vi "Tx Disable channel logic 4ch 4SPC.vi"(5 "num channels":u32, 6 "ready for output":bool, 9 "input valid":bool, 10 "data in":u32[](array[numeric])=[0, 0, 0, 0, 0, 0, 0, 0, 0, 0, 0, 0, 0, 0, 0, 0], 11 "enabled channels":u32) -> (0 "enable new data":bool, 1 "output valid":bool, 2 "data out":u32[](array[numeric]))   [LabVIEW 2025, in "niUSRP Stream Control (DMA) v1 FPGA.lvclass"]
uses:
  niUSRP Stream Control (DMA) v1 FPGA.lvclass
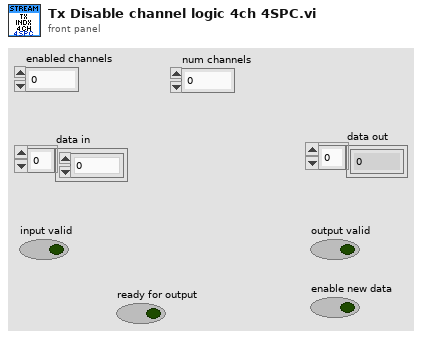
[diagram p1: front panel]
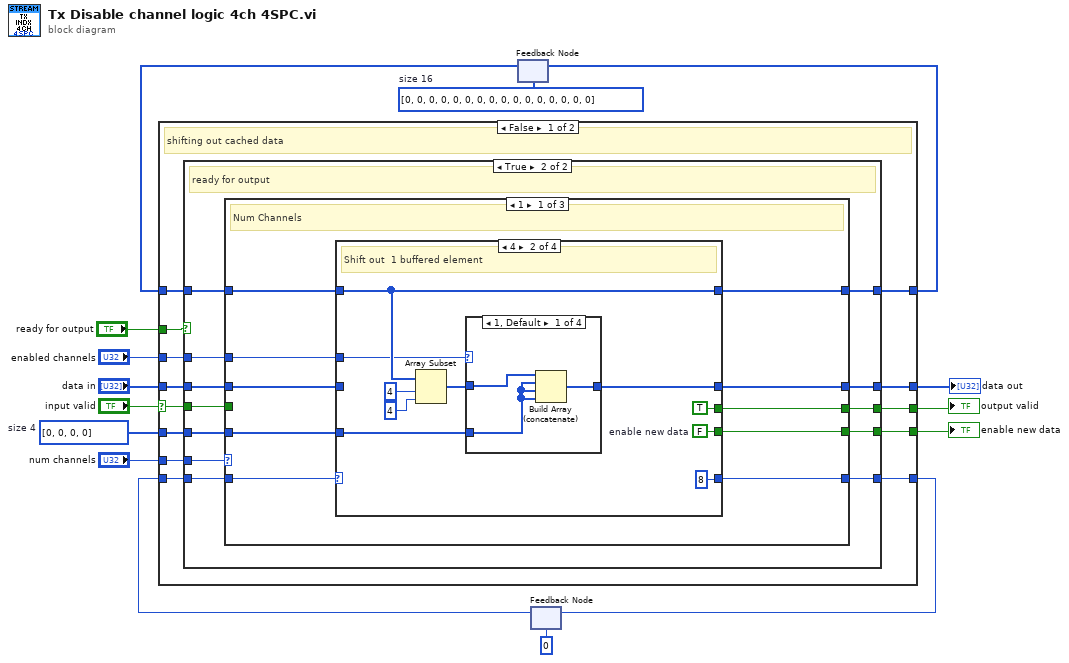
[diagram p0: block diagram]
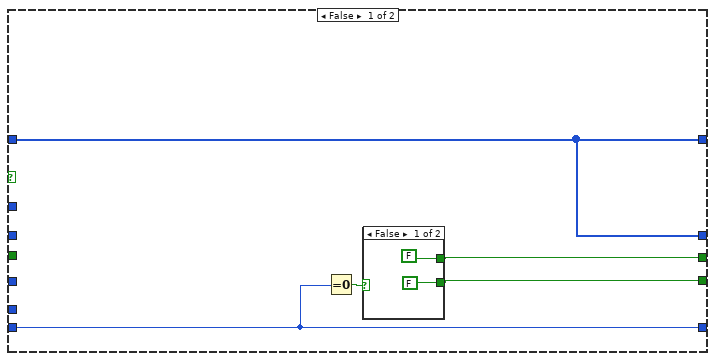
[diagram p2: hidden frame]
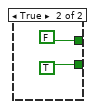
[diagram p3: hidden frame]
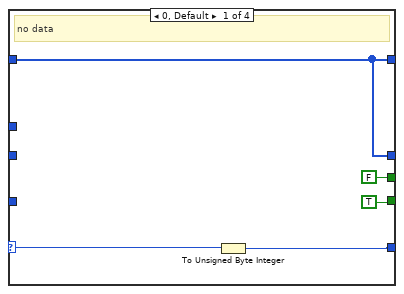
[diagram p4: hidden frame]
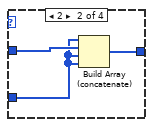
[diagram p5: hidden frame]
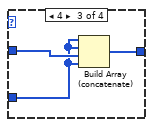
[diagram p6: hidden frame]
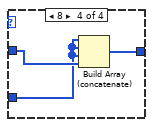
[diagram p7: hidden frame]
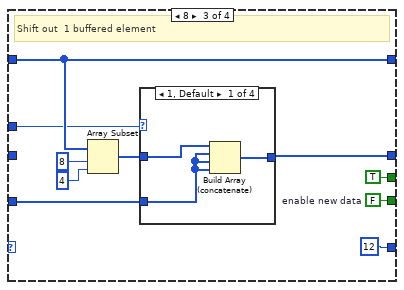
[diagram p8: hidden frame]
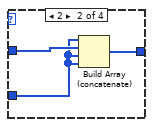
[diagram p9: hidden frame]
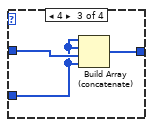
[diagram p10: hidden frame]
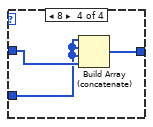
[diagram p11: hidden frame]
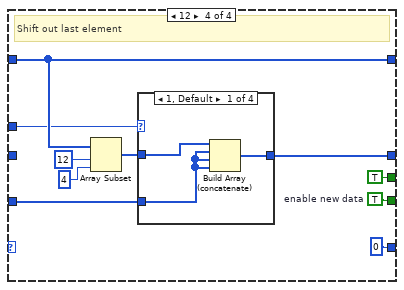
[diagram p12: hidden frame]
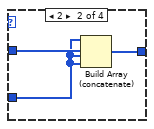
[diagram p13: hidden frame]
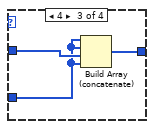
[diagram p14: hidden frame]
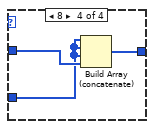
[diagram p15: hidden frame]
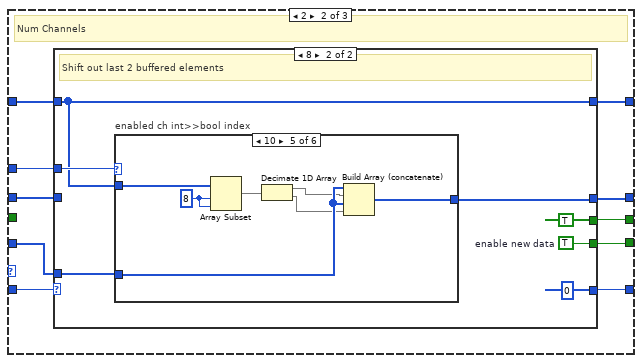
[diagram p16: hidden frame]
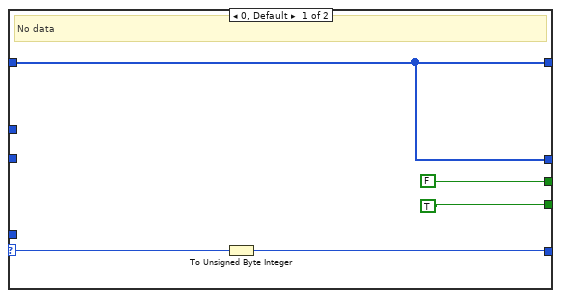
[diagram p17: hidden frame]
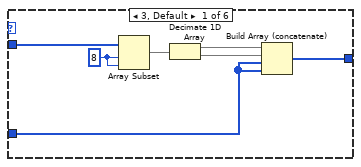
[diagram p18: hidden frame]
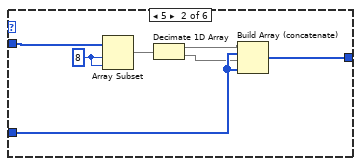
[diagram p19: hidden frame]
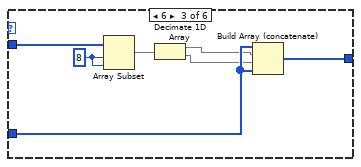
[diagram p20: hidden frame]
diagram:
  w2 = u32[] [0, 0, 0, 0]  # size 4
  w7 = u32[] [0, 0, 0, 0, 0, 0, 0, 0, 0, 0, 0, 0, 0, 0, 0, 0]  # size 16
  n1 = feedback #1(w7) -> (w6:u32[])
  n2 = feedback #2(u8 0) -> (w3:u8)
  n3 = case shown="False" "input valid" {
    selector: "input valid" -> [w19 _]
    tunnel: "num channels" -> [w28 w211]
    tunnel: [w27 w207] -> w14
    tunnel: [w26 w206] -> w13
    tunnel: "data in" -> [w25 w208]
    tunnel: "enabled channels" -> [w24 w203]
    tunnel: [w23 w205] -> w10
    tunnel: w6 -> [w22 w202]
    tunnel: [w21 w204] -> w5
    tunnel: [w16 w210] -> w4
    tunnel: w3 -> [w20 w209]
    tunnel: w2 -> [w18 w201]
    tunnel: "ready for output" -> [w17 _]
    frame False {
      # "shifting out cached data"
      n4 = case shown="True" w17 {
        tunnel: w28 -> [_ w49]
        tunnel: [w31 w48] -> w27
        tunnel: [w30 w47] -> w26
        tunnel: w25 -> [_ w46]
        tunnel: w24 -> [_ w45]
        tunnel: [w29 w44] -> w23
        tunnel: w22 -> [w29 w43]
        tunnel: [w29 w42] -> w21
        tunnel: w20 -> [w32 w41]
        tunnel: w19 -> [_ w39]
        tunnel: w18 -> [_ w38]
        tunnel: [w32 w40] -> w16
        frame False {
          n5 = Equal To 0?(x=w32) -> (x = 0?=w33:bool)
          n6 = case shown="False" w33 {
            tunnel: [FALSE TRUE] -> w30
            tunnel: [FALSE FALSE] -> w31
            frame False {
            }
            frame True {
            }
          }
        }
        frame True {
          # "ready for output"
          n7 = case shown="1" w49 {
            tunnel: w45 -> [w59 w139 _]
            tunnel: w46 -> [w58 w140 w200]
            tunnel: [w57 w136 w199] -> w47
            tunnel: [w56 w137 w196] -> w48
            tunnel: [w55 w138 w200] -> w44
            tunnel: w43 -> [w51 w132 w197]
            tunnel: [w54 w133 w197] -> w42
            tunnel: w41 -> [w53 w134 w198]
            tunnel: [w52 w135 w195] -> w40
            tunnel: w39 -> [_ _ w196]
            tunnel: w38 -> [w50 w131 _]
            frame 1 {
              # "Num Channels"
              n8 = case shown="4" w53 {
                selector: w53 -> [w61 _ _ _]
                tunnel: w58 -> [_ _ _ _]
                tunnel: [w60 u8 8 ("length") u8 12 ("length") u8 0] -> w52
                tunnel: [w62 w65 w96 w113] -> w55
                tunnel: [FALSE TRUE TRUE TRUE] -> w56
                tunnel: w51 -> [w62 w73 w94 w115]
                tunnel: [w62 w73 w94 w115] -> w54
                tunnel: [TRUE w72 w93 w116] -> w57
                tunnel: w59 -> [_ w67 w92 w112]
                tunnel: w50 -> [_ w68 w90 w111]
                frame 0, Default {
                  # "no data"
                  n9 = To Unsigned Byte Integer(number=w61) -> (unsigned 8bit integer=w60:u8)
                }
                frame 4 {
                  w72 = FALSE  # enable new data
                  # "Shift out  1 buffered element"
                  n10 = Array Subset(array=w73, index=i16 4 ("length"), length=i16 4) -> (w66:u32[])
                  n11 = case shown="1, Default" w67 {
                    tunnel: [w77 w80 w83 w86] -> w65
                    tunnel: w66 -> [w76 w79 w82 w85]
                    tunnel: w68 -> [w75 w78 w81 w84]
                    frame 1, Default {
                      n12 = Build Array (concatenate)(w76, w75, w75, w75) -> (w77:u32[])
                    }
                    frame 2 {
                      n13 = Build Array (concatenate)(w78, w79, w78, w78) -> (w80:u32[])
                    }
                    frame 4 {
                      n14 = Build Array (concatenate)(w81, w81, w82, w81) -> (w83:u32[])
                    }
                    frame 8 {
                      n15 = Build Array (concatenate)(w84, w84, w84, w85) -> (w86:u32[])
                    }
                  }
                }
                frame 8 {
                  w93 = FALSE  # enable new data
                  # "Shift out  1 buffered element"
                  n16 = Array Subset(array=w94, index=i16 8 ("length"), length=i16 4) -> (w91:u32[])
                  n17 = case shown="1, Default" w92 {
                    tunnel: [w99 w102 w105 w108] -> w96
                    tunnel: w91 -> [w98 w101 w104 w107]
                    tunnel: w90 -> [w97 w100 w103 w106]
                    frame 1, Default {
                      n18 = Build Array (concatenate)(w98, w97, w97, w97) -> (w99:u32[])
                    }
                    frame 2 {
                      n19 = Build Array (concatenate)(w100, w101, w100, w100) -> (w102:u32[])
                    }
                    frame 4 {
                      n20 = Build Array (concatenate)(w103, w103, w104, w103) -> (w105:u32[])
                    }
                    frame 8 {
                      n21 = Build Array (concatenate)(w106, w106, w106, w107) -> (w108:u32[])
                    }
                  }
                }
                frame 12 {
                  w116 = TRUE  # enable new data
                  # "Shift out last element"
                  n22 = Array Subset(array=w115, index=12, length=4) -> (w109:u32[])
                  n23 = case shown="1, Default" w112 {
                    tunnel: [w121 w124 w127 w130] -> w113
                    tunnel: w109 -> [w120 w123 w126 w129]
                    tunnel: w111 -> [w119 w122 w125 w128]
                    frame 1, Default {
                      n24 = Build Array (concatenate)(w120, w119, w119, w119) -> (w121:u32[])
                    }
                    frame 2 {
                      n25 = Build Array (concatenate)(w122, w123, w122, w122) -> (w124:u32[])
                    }
                    frame 4 {
                      n26 = Build Array (concatenate)(w125, w125, w126, w125) -> (w127:u32[])
                    }
                    frame 8 {
                      n27 = Build Array (concatenate)(w128, w128, w128, w129) -> (w130:u32[])
                    }
                  }
                }
              }
            }
            frame 2 {
              # "Num Channels"
              n28 = case shown="8" w134 {
                selector: w134 -> [w142 _]
                tunnel: w140 -> [_ _]
                tunnel: [w141 u8 0] -> w135
                tunnel: [w143 w148] -> w138
                tunnel: [FALSE TRUE] -> w137
                tunnel: w132 -> [w143 w146]
                tunnel: [w143 w146] -> w133
                tunnel: [TRUE w150] -> w136
                tunnel: w139 -> [_ w149]
                tunnel: w131 -> [_ w147]
                frame 0, Default {
                  # "No data"
                  n29 = To Unsigned Byte Integer(number=w142) -> (unsigned 8bit integer=w141:u8)
                }
                frame 8 {
                  w150 = TRUE  # enable new data
                  # "Shift out last 2 buffered elements"
                  n30 = case "enabled ch int>>bool index" shown="10" w149 {
                    tunnel: [w159 w166 w173 w180 w187 w194] -> w148
                    tunnel: w147 -> [w158 w165 w172 w179 w186 w193]
                    tunnel: w146 -> [w156 w162 w169 w176 w183 w190]
                    frame 3, Default {
                      w155 = 8 ("index")
                      n31 = Array Subset(array=w156, index=w155, length=w155) -> (w157:u32[])
                      n32 = Decimate 1D Array(w157) -> (w154:u32[], w153:u32[])
                      n33 = Build Array (concatenate)(w154, w153, w158, w158) -> (w159:u32[])
                    }
                    frame 5 {
                      w163 = 8 ("index")
                      n34 = Array Subset(array=w162, index=w163, length=w163) -> (w164:u32[])
                      n35 = Decimate 1D Array(w164) -> (w161:u32[], w160:u32[])
                      n36 = Build Array (concatenate)(w161, w165, w160, w165) -> (w166:u32[])
                    }
                    frame 6 {
                      w170 = 8 ("index")
                      n37 = Array Subset(array=w169, index=w170, length=w170) -> (w171:u32[])
                      n38 = Decimate 1D Array(w171) -> (w168:u32[], w167:u32[])
                      n39 = Build Array (concatenate)(w172, w168, w167, w172) -> (w173:u32[])
                    }
                    frame 9 {
                      w177 = 8 ("index")
                      n40 = Array Subset(array=w176, index=w177, length=w177) -> (w178:u32[])
                      n41 = Decimate 1D Array(w178) -> (w175:u32[], w174:u32[])
                      n42 = Build Array (concatenate)(w175, w179, w179, w174) -> (w180:u32[])
                    }
                    frame 10 {
                      w184 = 8 ("index")
                      n43 = Array Subset(array=w183, index=w184, length=w184) -> (w185:u32[])
                      n44 = Decimate 1D Array(w185) -> (w182:u32[], w181:u32[])
                      n45 = Build Array (concatenate)(w186, w182, w186, w181) -> (w187:u32[])
                    }
                    frame 12 {
                      w191 = 8 ("index")
                      n46 = Array Subset(array=w190, index=w191, length=w191) -> (w192:u32[])
                      n47 = Decimate 1D Array(w192) -> (w189:u32[], w188:u32[])
                      n48 = Build Array (concatenate)(w193, w193, w189, w188) -> (w194:u32[])
                    }
                  }
                }
              }
            }
            frame 4, Default {
              w199 = TRUE  # enable new data
              # "Num Channels"
              n49 = To Unsigned Byte Integer(number=w198) -> (unsigned 8bit integer=w195:u8)
            }
          }
        }
      }
    }
    frame True {
      # "input valid >>cache data"
      n50 = case shown="1, Default" w211 {
        tunnel: [u8 4 ("x") u8 8 ("length") u8 0 ("length")] -> w210
        tunnel: w209 -> [_ _ _]
        tunnel: w208 -> [w217 w234 w290]
        tunnel: [TRUE TRUE TRUE] -> w207
        tunnel: [w220 FALSE ("enable new data") w297] -> w206
        tunnel: [w212 w235 w289] -> w205
        tunnel: [w217 w234 w295] -> w204
        tunnel: w203 -> [w215 w237 _]
        tunnel: w202 -> [_ _ w295]
        tunnel: w201 -> [w213 w236 _]
        frame 1, Default {
          w220 = FALSE  # enable new data
          # "Send data to enabled channel\nRemaining 3 channels set to default \"0\""
          # "Grab data for \n1ch - 4SPC"
          # "Num Enabled Channels"
          n51 = Array Subset(array=w217, index=0, length=4) -> (w214:u32[])
          n52 = case shown="1, Default" w215 {
            tunnel: [w224 w227 w230 w233] -> w212
            tunnel: w213 -> [w223 w226 w229 w232]
            tunnel: w214 -> [w222 w225 w228 w231]
            frame 1, Default {
              # "enabled ch int>>bool index"
              n53 = Build Array (concatenate)(w222, w223, w223, w223) -> (w224:u32[])
            }
            frame 2 {
              # "enabled ch int>>bool index"
              n54 = Build Array (concatenate)(w226, w225, w226, w226) -> (w227:u32[])
            }
            frame 4 {
              # "enabled ch int>>bool index"
              n55 = Build Array (concatenate)(w229, w229, w228, w229) -> (w230:u32[])
            }
            frame 8 {
              # "enabled ch int>>bool index"
              n56 = Build Array (concatenate)(w232, w232, w232, w231) -> (w233:u32[])
            }
          }
        }
        frame 2 {
          # "Grab 2 channels\ninterleaved data\n(0,1,0,1,0,1,0,1..)"
          # "Num Enabled Channels"
          n57 = case "enabled ch int>>bool index" shown="3, Default" w237 {
            tunnel: [w248 w256 w264 w272 w280 w288] -> w235
            tunnel: w236 -> [w247 w255 w263 w271 w279 w287]
            tunnel: w234 -> [w245 w251 w259 w267 w275 w283]
            frame 3, Default {
              n58 = Array Subset(array=w245, index=0 ("y"), length=8 ("y")) -> (w246:u32[])
              n59 = Decimate 1D Array(w246) -> (w242:u32[], w241:u32[])
              n60 = Build Array (concatenate)(w242, w241, w247, w247) -> (w248:u32[])
            }
            frame 5 {
              n61 = Array Subset(array=w251, index=0 ("y"), length=8 ("y")) -> (w254:u32[])
              n62 = Decimate 1D Array(w254) -> (w250:u32[], w249:u32[])
              n63 = Build Array (concatenate)(w250, w255, w249, w255) -> (w256:u32[])
            }
            frame 6 {
              n64 = Array Subset(array=w259, index=0 ("y"), length=8 ("y")) -> (w262:u32[])
              n65 = Decimate 1D Array(w262) -> (w258:u32[], w257:u32[])
              n66 = Build Array (concatenate)(w263, w258, w257, w263) -> (w264:u32[])
            }
            frame 9 {
              n67 = Array Subset(array=w267, index=0 ("y"), length=8 ("y")) -> (w270:u32[])
              n68 = Decimate 1D Array(w270) -> (w266:u32[], w265:u32[])
              n69 = Build Array (concatenate)(w266, w271, w271, w265) -> (w272:u32[])
            }
            frame 10 {
              n70 = Array Subset(array=w275, index=0 ("y"), length=8 ("y")) -> (w278:u32[])
              n71 = Decimate 1D Array(w278) -> (w274:u32[], w273:u32[])
              n72 = Build Array (concatenate)(w279, w274, w279, w273) -> (w280:u32[])
            }
            frame 12 {
              n73 = Array Subset(array=w283, index=0 ("y"), length=8 ("y")) -> (w286:u32[])
              n74 = Decimate 1D Array(w286) -> (w282:u32[], w281:u32[])
              n75 = Build Array (concatenate)(w287, w287, w282, w281) -> (w288:u32[])
            }
          }
        }
        frame 4 {
          w297 = TRUE  # enable new data
          # "Data from driver is interleaved (0,1,2,3,0,1,2,3....)\nDSP needs data in grouping of 4SPC (0,0,0,0,1,1,1,1...)"
          # "Num Enabled Channels"
          n76 = Decimate 1D Array(w290) -> (w294:u32[], w293:u32[], w292:u32[], w291:u32[])
          n77 = Build Array (concatenate)(w294, w293, w292, w291) -> (w289:u32[])
        }
      }
    }
  }
  "output valid" <- w14
  "enable new data" <- w13
  "data out" <- w10
  n78 = feedback-in #1(w5) -> ()
  n79 = feedback-in #2(w4) -> ()
